vi "RIF_RII.vi"() -> ()   [LabVIEW 2018]
uses:
  <vilib>/measure/maspectr.llb/FFT Spectrum (Mag-Phase) for 1 Chan.vi
  <vilib>/measure/macond.llb/IIR Filter for 1 Chan.vi
  <vilib>/measure/macond.llb/FIR Filter for 1 Chan.vi
  <vilib>/measure/NI_MABase.lvlib
  <vilib>/Analysis/NI_AALBase.lvlib
  <vilib>/measure/NI_MAPro.lvlib
panel:
  out "siganl par RIF":waveform(dbl)(graph)
  out "siganl par RII":waveform(dbl)(graph)
  out "Spectre signal filtre par RIF":cluster{"f0":dbl, "df":dbl, "Mag H(w)":dbl[]}(graph)
  out "Spectre filtré par RII":cluster{"f0":dbl, "df":dbl, "Mag H(w)":dbl[]}(graph)
  out "Spectre avant filtrage":cluster{"f0":dbl, "df":dbl, "Mag H(w)":dbl[]}(graph)
  out "Gain filtre RIF":cluster{"f0":dbl, "df":dbl, "Mag H(w)":dbl[]}(graph)
  in  "FIR filter specifications":T1={"Topology"=enum."Off", "Type"=enum."Lowpass", "#Taps"=50, "Lower PB"=100.0, "Upper PB"=0.0, "Lower SB"=200.0, "Upper SB"=0.0} {"Lower SB" format="%0.2p"; "Upper SB" format="%0.2p"; "Lower PB" format="%0.2p"; "Upper PB" format="%0.2p"}
  in  "IIR filter specifications":T2={"Topology"=enum."Butterworth", "Type"=enum."Lowpass", "Order"=1, "Lower Fc"=100.0, "Upper Fc"=200.0, "PB Ripple"=1.0, "SB Attenuation"=60.0} {"PB Ripple" format="%0.2f"; "SB Attenuation" format="%0.2f"; "Lower Fc" format="%0.2p"; "Upper Fc" format="%0.2p"}
  out "Gain filtre RII":cluster{"f0":dbl, "df":dbl, "Mag H(w)":dbl[]}(graph)
  out "Waveform Graph":waveform(dbl)(graph)
  in  "Ampli Bruit":dbl=1.0 format="%0.2f"
  in  "Boolean":bool
  in  "signal type":T3(ring)
  in  "amplitude":dbl=1.0 format="%0.2p"
  in  "frequency":dbl=10.0 format="%0.2p"
  in  "nbre N":i32=2
  in  "stop":bool
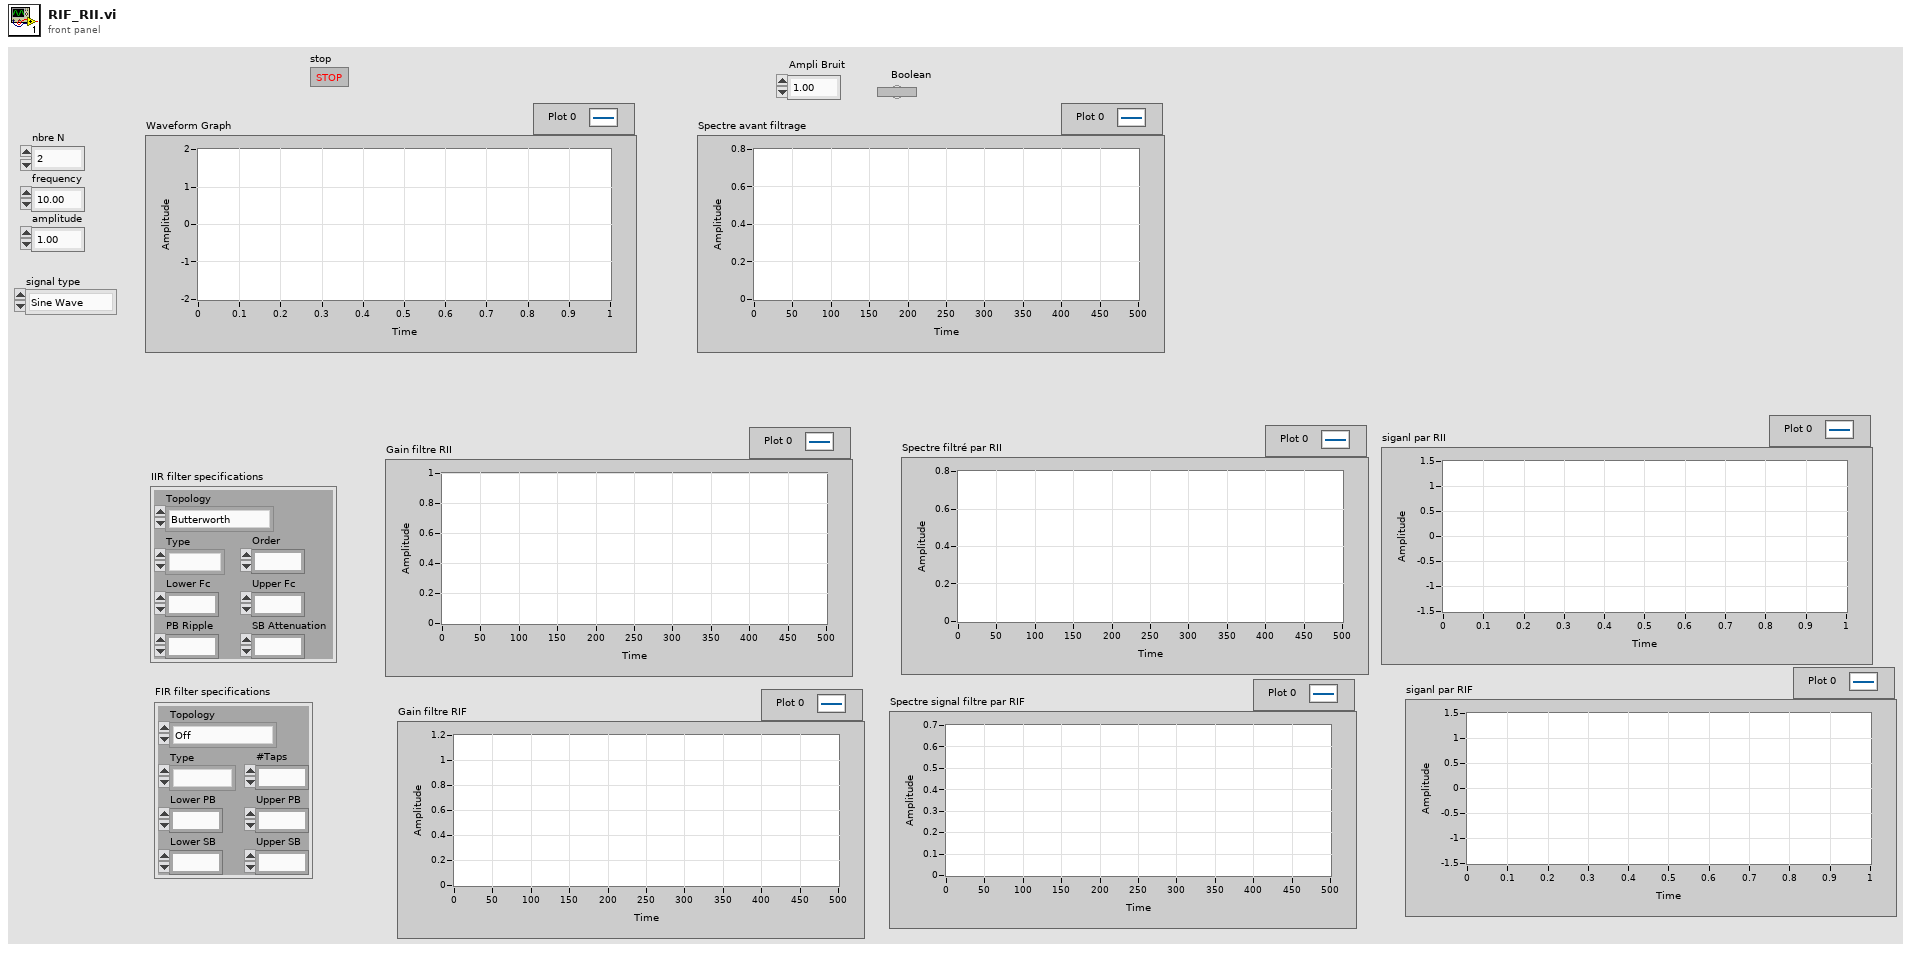
[diagram p1: front panel]
types:
  T1 = cluster{"Topology":enum16{"Off", "FIR by Specification", "Equi-ripple FIR", "Windowed FIR"}, "Type":enum16{"Lowpass", "Highpass", "Bandpass", "Bandstop"}, "#Taps":i32, "Lower PB":dbl, "Upper PB":dbl, "Lower SB":dbl, "Upper SB":dbl}
  T2 = cluster{"Topology":enum16{"Off", "Butterworth", "Chebyshev", "Inverse Chebyshev", "Elliptic", "Bessel"}, "Type":enum16{"Lowpass", "Highpass", "Bandpass", "Bandstop"}, "Order":i32, "Lower Fc":dbl, "Upper Fc":dbl, "PB Ripple":dbl, "SB Attenuation":dbl}
  T3 = enum16{"Sine Wave", "Triangle Wave", "Square Wave", "Sawtooth Wave"}
  T4 = cluster{"magnitude H(w)":cluster{"f0":dbl, "df":dbl, "Mag H(w)":dbl[]}, "phase H(w)":cluster{"f0":dbl, "df":dbl, "Phase H(w)":dbl[]}, "order":i32}
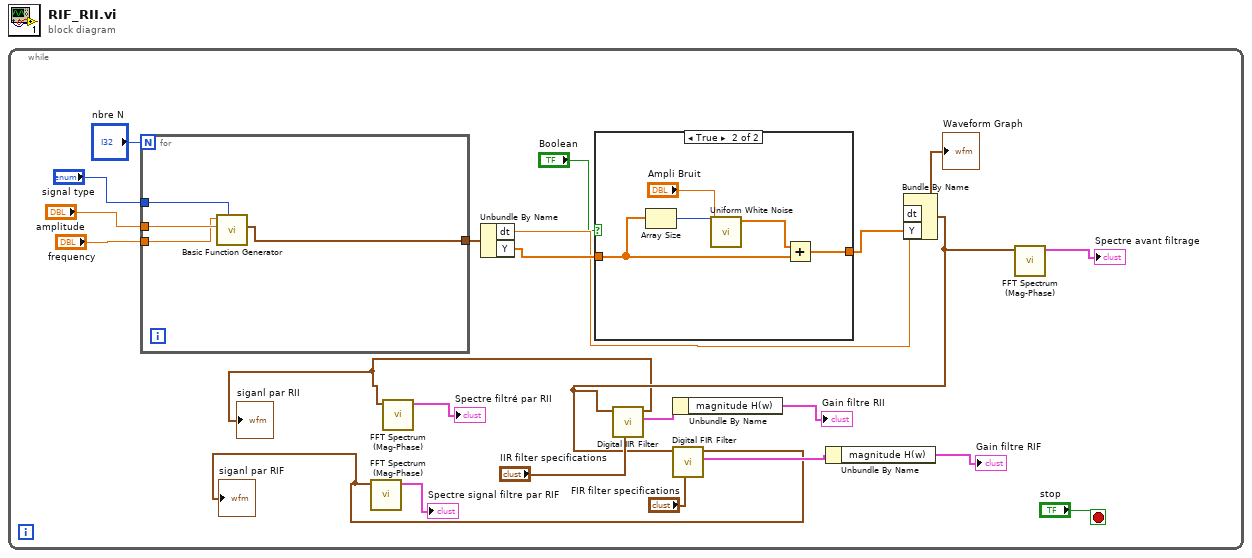
[diagram p0: block diagram]
diagram:
  n1 = while {
    stop <- "stop" stop-if-true
    n2 = for {
      N: "nbre N" -> [_]
      tunnel: "signal type" -> [w32]
      tunnel: "amplitude" -> [w31]
      tunnel: "frequency" -> [w30]
      tunnel: [w29] -> w16
      n3 = call <vilib>:"Basic Function Generator.vi"("signal type"=w32, "amplitude"=w31, "frequency"=w30) -> ("signal out"=w29:waveform(dbl))  [unwired: 6 in, 2 out]
    }
    n4 = Unbundle By Name(w16) -> ("dt"=w14:dbl, "Y"=w17:dbl[])
    n5 = case shown="True" "Boolean" {
      tunnel: w17 -> [w23 w24]
      tunnel: [w23 w25] -> w15
      frame False {
      }
      frame True {
        n6 = Array Size(array=w24) -> (size(s)=w28:i32)
        n7 = call <vilib>:"Uniform White Noise.vi"("amplitude"="Ampli Bruit", "samples"=w28) -> ("uniform white noise"=w26:dbl[])  [unwired: 8 in, 1 out]
        n8 = Add(x=w26, y=w24) -> (x+y=w25:dbl[])
      }
    }
    n9 = Bundle By Name("dt"=w14, "Y"=w15) -> (w6:waveform(dbl))  [unwired: 1 in]
    "Waveform Graph" <- w6
    n10 = call-poly <vilib>:"Digital IIR Filter.vi"("IIR filter specifications"="IIR filter specifications", "signal in"=w6) -> ("filter information"=w11:T4, "signal out"=w1:waveform(dbl))  [unwired: 7 in, 1 out]
    "siganl par RII" <- w1
    n11 = call-poly <vilib>:"FFT Spectrum (Mag-Phase).vi"("time signal"=w1) -> ("magnitude"=→"Spectre filtré par RII":cluster{"f0":dbl, "df":dbl, "magnitude":dbl[]})  [unwired: 6 in, 4 out]
    n12 = Unbundle By Name(w11) -> ("magnitude H(w)"=→"Gain filtre RII":cluster{"f0":dbl, "df":dbl, "Mag H(w)":dbl[]})
    n13 = call-poly <vilib>:"Digital FIR Filter.vi"("FIR filter specifications"="FIR filter specifications", "signal in"=w6) -> ("filter information"=w12:T4, "signal out"=w2:waveform(dbl))  [unwired: 7 in, 1 out]
    "siganl par RIF" <- w2
    n14 = call-poly <vilib>:"FFT Spectrum (Mag-Phase).vi"("time signal"=w2) -> ("magnitude"=→"Spectre signal filtre par RIF":cluster{"f0":dbl, "df":dbl, "magnitude":dbl[]})  [unwired: 6 in, 4 out]
    n15 = Unbundle By Name(w12) -> ("magnitude H(w)"=→"Gain filtre RIF":cluster{"f0":dbl, "df":dbl, "Mag H(w)":dbl[]})
    n16 = call-poly <vilib>:"FFT Spectrum (Mag-Phase).vi"("time signal"=w6) -> ("magnitude"=→"Spectre avant filtrage":cluster{"f0":dbl, "df":dbl, "magnitude":dbl[]})  [unwired: 6 in, 4 out]
  }
